vi "Example Simple.vi"() -> ()   [LabVIEW 2013]
uses:
  C:/tf/play/labview/Tinkerforge.dll
panel:
  out "tilt state":string
  in  "uid":string="gfdd"
  in  "port":i32=4223
  in  "host":string="localhost"
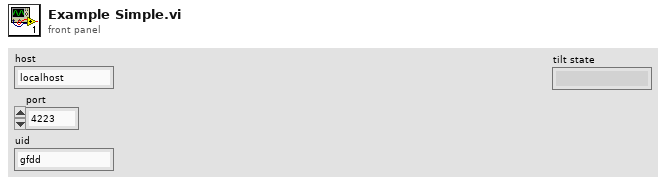
[diagram p1: front panel]
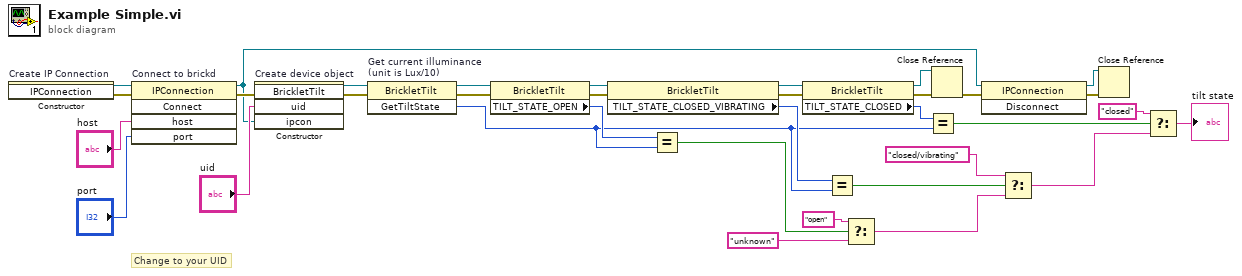
[diagram p0: block diagram]
diagram:
  # "Change to your UID"
  n1 = constructor on="Create IP Connection" class="IPConnection"() -> (reference out=w34:refnum<k24>, error out=w23:errorcluster)  [unwired: 3 in, 1 out]
  n2 = invoke on="Connect to brickd" class="IPConnection" method="Connect"(reference=w34, error in=w23, "host"="host", "port"="port") -> (reference out=w25:refnum<k24>, error out=w30:errorcluster)  [unwired: 1 in, 3 out]
  n3 = constructor on="Create device object" class="BrickletTilt"(error in=w30, "uid"="uid", "ipcon"=w25) -> (reference out=w28:refnum<k24>, error out=w29:errorcluster)  [unwired: 2 in, 3 out]
  n4 = invoke on="Get current illuminance\n(unit is Lux/10)" class="BrickletTilt" method="GetTiltState"(reference=w28, error in=w29) -> (reference out=w6:refnum<k24>, error out=w4:errorcluster, "GetTiltState"=w5:u8)  [unwired: 1 in]
  n5 = property class="BrickletTilt"(reference=w6, error in=w4) -> (reference out=w13:refnum<k24>, error out=w12:errorcluster, "TILT_STATE_OPEN"=w11:u8)
  n6 = property class="BrickletTilt"(reference=w13, error in=w12) -> (reference out=w19:refnum<k24>, error out=w18:errorcluster, "TILT_STATE_CLOSED_VIBRATING"=w15:u8)
  n7 = Equal?(x=w11, y=w5) -> (x = y?=w10:bool)
  n8 = property class="BrickletTilt"(reference=w19, error in=w18) -> (reference out=w1:refnum<k24>, error out=w2:errorcluster, "TILT_STATE_CLOSED"=w22:u8)
  n9 = Equal?(x=w15, y=w5) -> (x = y?=w17:bool)
  n10 = Select(t="open", s=w10, f="unknown") -> (s? t:f=w7:string)
  n11 = Equal?(x=w22, y=w5) -> (x = y?=w21:bool)
  n12 = Close Reference(reference=w1, error in (no error)=w2) -> (error out=w27:errorcluster)
  n13 = invoke class="IPConnection" method="Disconnect"(reference=w25, error in=w27) -> (reference out=w24:refnum<k24>, error out=w26:errorcluster)  [unwired: 1 in, 1 out]
  n14 = Select(t="closed/vibrating", s=w17, f=w7) -> (s? t:f=w14:string)
  n15 = Close Reference(reference=w24, error in (no error)=w26) -> ()  [unwired: 1 out]
  n16 = Select(t="closed", s=w21, f=w14) -> (s? t:f=→"tilt state":string)
